vi "Initialize.vi"(8 "error in":errorcluster, 9 "parameters":variant, 10 "path":path, 11 "repository in":refnum<class "NISE_CEF_Repository.lvclass">) -> (0 "error out":errorcluster, 3 "repository out":refnum<class "NISE_CEF_Repository.lvclass">)   [LabVIEW 2013, in "NISE_CEF_Repository.lvclass"]
doc: "Initializes the repo. StoreClassPath method should be called in this VI"
uses:
  NISE_CEF_Repository.lvclass
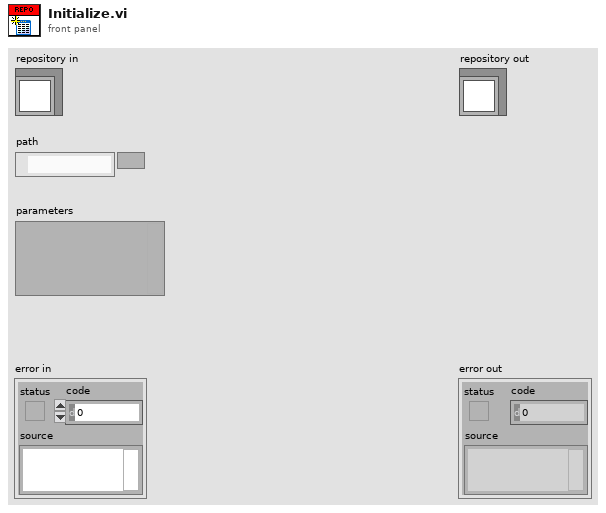
[diagram p1: front panel]
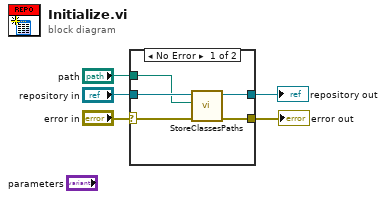
[diagram p0: block diagram]
diagram:
  n1 = case shown="No Error" "error in" {
    selector: "error in" -> [w8 w12]
    tunnel: [w7 w12] -> w4
    tunnel: [w9 w11] -> w2
    tunnel: "repository in" -> [w10 w11]
    tunnel: "path" -> [w6 _]
    frame No Error {
      n2 = call-dynamic "StoreClassesPaths.vi"("error in"=w8, "start path"=w6, "Repository in"=w10) -> ("error out"=w7:errorcluster, "Repository out"=w9:refnum<class "NISE_CEF_Repository.lvclass">)  [unwired: 7 in]
    }
    frame Error {
    }
  }
  "error out" <- w4
  "repository out" <- w2
